vi "solenoid-sample.vi"() -> ()   [LabVIEW 2020]
uses:
  <vilib>/Rock Robotics/SystemInterfaces/DIO/FPGA_DIORelayChannel.ctl
  <vilib>/Rock Robotics/WPI/Relay/WPI_RelayDirection.ctl
  <vilib>/Rock Robotics/WPI/Relay/WPI_RelayValue.ctl
  <vilib>/Rock Robotics/WPI/Solenoid/WPI_SolenoidChannel.ctl
  <vilib>/Rock Robotics/WPI/Solenoid/WPI_SolenoidValue.ctl
  <vilib>/Rock Robotics/WPI/ThirdParty/JAS_Junk/TrajLib/Timer_New.vi
  <vilib>/Rock Robotics/WPI/Utilities/WPI_GetSetVariantRefNum.vi
  <vilib>/Rock Robotics/Network Tables/NT Write Boolean.vi
  <vilib>/Rock Robotics/Network Tables/NT Write Number.vi
  <vilib>/Rock Robotics/WPI/Solenoid/WPI_SolenoidOpenSingle.vi
  <vilib>/Rock Robotics/WPI/Solenoid/WPI_SolenoidOpenDouble.vi
  <vilib>/Rock Robotics/WPI/Solenoid/WPI_SolenoidSetEnum.vi
  <vilib>/Utility/semaphor.llb/Obtain Semaphore Reference.vi
  <vilib>/Rock Robotics/WPI/ThirdParty/JAS_Junk/TrajLib/Timer_Reset.vi
  <vilib>/Rock Robotics/WPI/ThirdParty/JAS_Junk/TrajLib/Timer_Start.vi
  <vilib>/Rock Robotics/WPI/ThirdParty/JAS_Junk/TrajLib/Timer_HasPeriodPassedOnce.vi
  <vilib>/Rock Robotics/WPI/ThirdParty/JAS_Junk/TrajLib/Timer_Stop.vi
  <vilib>/Rock Robotics/Network Tables/NT Write Integer.vi
  <vilib>/Rock Robotics/WPI/ThirdParty/JAS_Junk/TrajLib/Trajectory_Library.lvlib
panel:
  in  "ROBOT\nENABLED":bool
  in  "SOLENOID\nCONTROL":bool
  in  "SOLENOID\nCONTROL":bool
  in  "RELAY\nREVERSE":bool
  in  "RELAY\nFORWARD":bool
  in  "RELAY\nCONTROL":bool
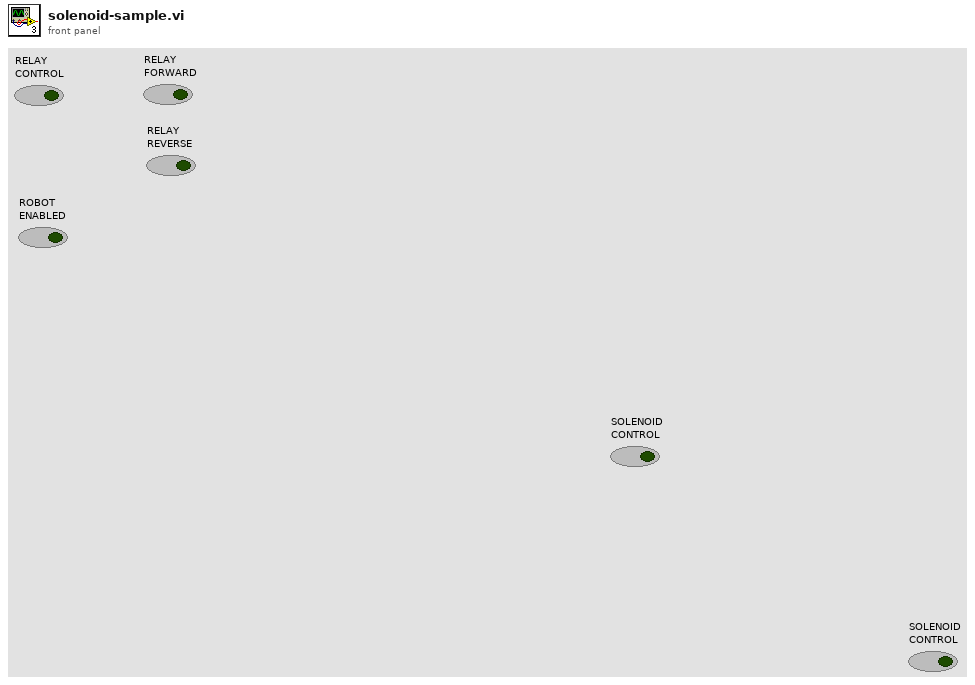
[diagram p1: front panel]
types:
  T1 = typedef "WPI_SolenoidValue.ctl" = enum16{"Off", "On", "Forward", "Reverse"}
  T2 = typedef "WPI_SolenoidChannel.ctl" = enum8{"Solenoid 0", "Solenoid 1", "Solenoid 2", "Solenoid 3", "Solenoid 4", "Solenoid 5", "Solenoid 6", "Solenoid 7", "Solenoid 8", "Solenoid 9", "Solenoid 10", "Solenoid 11", "Solenoid 12", "Solenoid 13", "Solenoid 14", "Solenoid 15", "Invalid"}
  T3 = typedef "WPI_RelayValue.ctl" = enum16{"Off", "On", "Forward", "Reverse"}
  T4 = typedef "WPI_RelayDirection.ctl" = enum16{"Both directions", "Forward only", "Reverse only"}
  T5 = typedef "FPGA_DIORelayChannel.ctl" = enum8{"Relay 0", "Relay 1", "Relay 2", "Relay 3", "Invalid"}
  T6 = typedef "WPI_CompressorDevRef.ctl" = cluster{"DevStatus":errorcluster, "Pneumatics Control Module":u8}
  T7 = typedef "WPI_RelayDevRef.ctl" = cluster{"DevStatus":errorcluster, "Relay Channel":T5, "Relay Direction":T4}
  T8 = typedef "WPI_SolenoidDevRef.ctl" = cluster{"DevStatus":errorcluster, "Pneumatics Control Module":u8, "Forward Solenoid Channel":T2, "Reverse Solenoid Channel":T2}
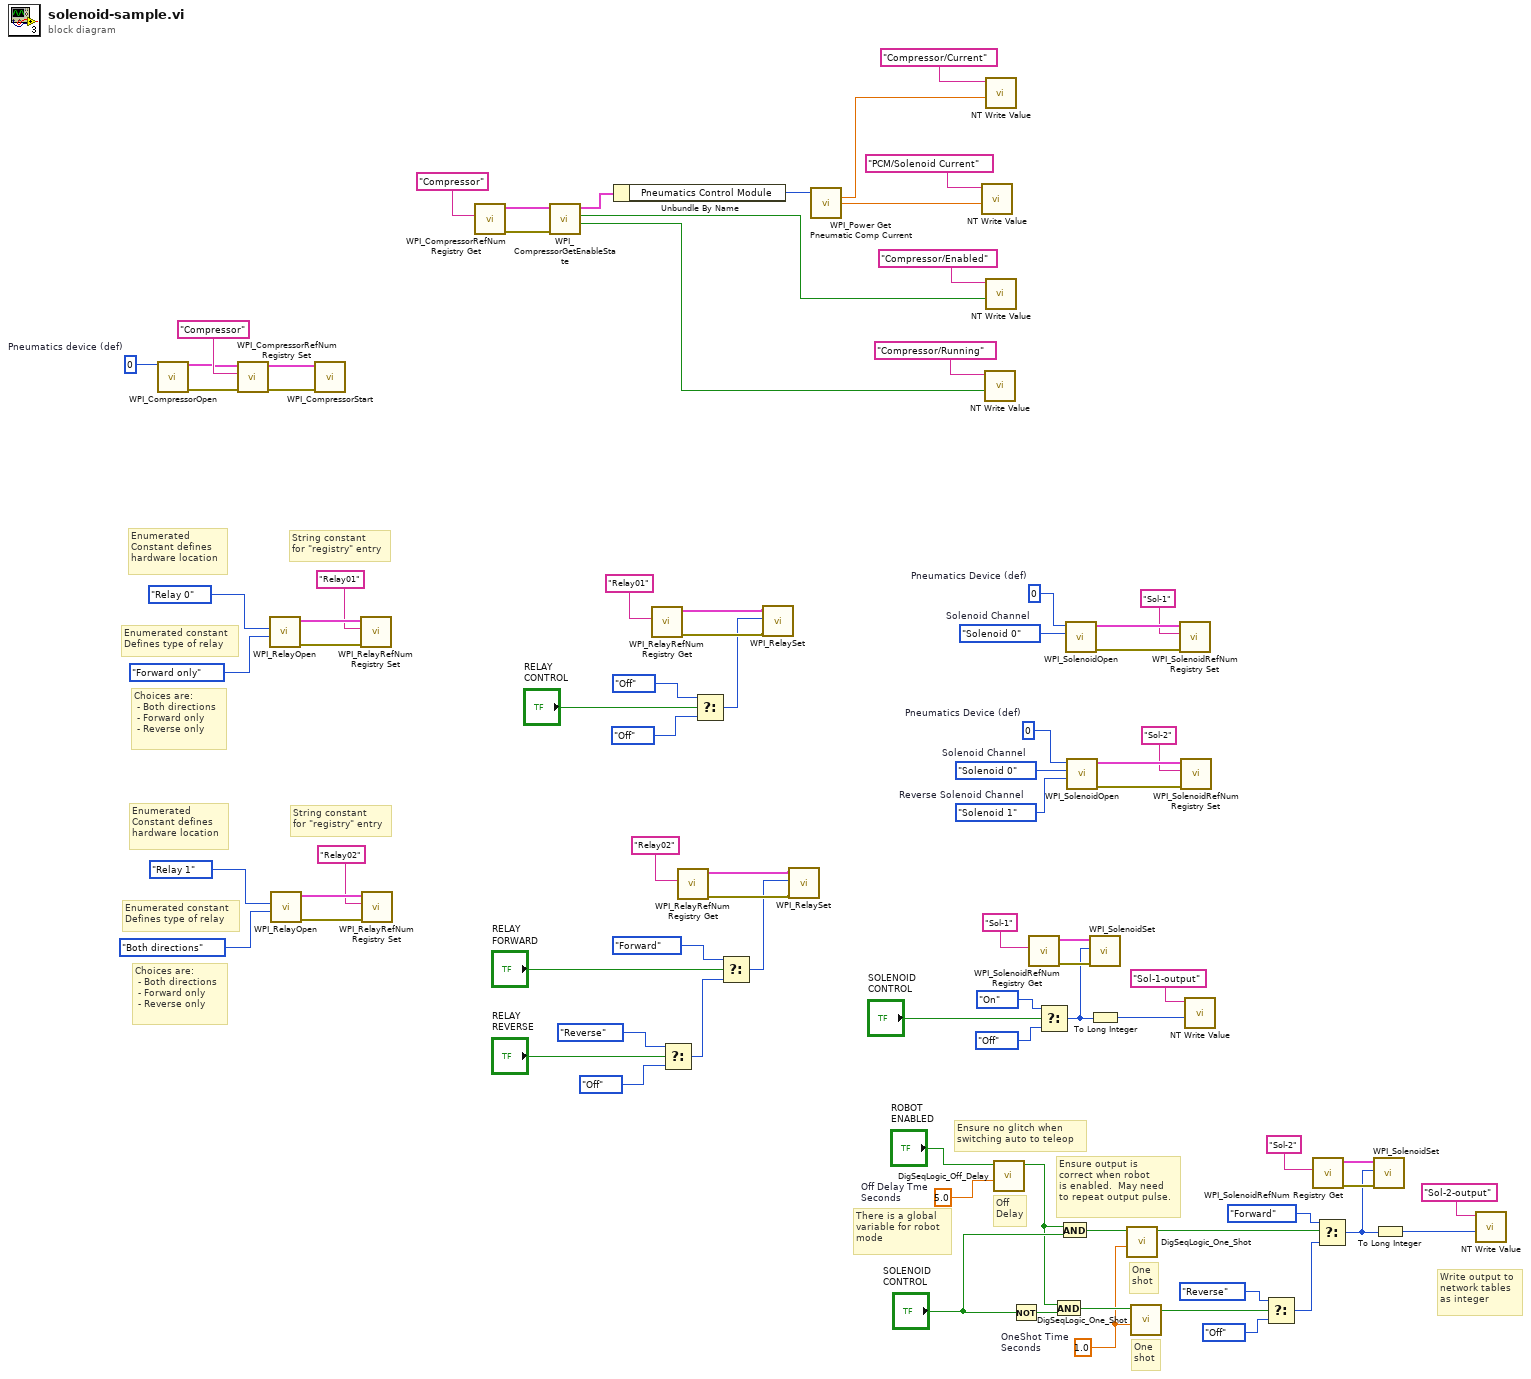
[diagram p0: block diagram]
diagram:
  w1 = 1.0  # OneShot Time Seconds
  w19 = 5.0  # Off Delay Tme Seconds
  w30 = WPI_SolenoidChannel."Solenoid 1"  # Reverse Solenoid Channel
  w31 = WPI_SolenoidChannel."Solenoid 0"  # Solenoid Channel
  w32 = u8 0  # Pneumatics Device (def)
  w36 = WPI_SolenoidChannel."Solenoid 0"  # Solenoid Channel
  w37 = u8 0  # Pneumatics Device (def)
  w59 = u8 0  # Pneumatics device (def)
  # "Ensure no glitch when\nswitching auto to teleop"
  # "There is a global \nvariable for robot \nmode"
  # "Write output to\nnetwork tables\nas integer"
  # "Ensure output is\ncorrect when robot\nis enabled.  May need\nto repeat output pulse."
  # "One \nshot"
  # "One \nshot"
  # "Off \nDelay"
  # "Choices are:\n - Both directions\n - Forward only\n - Reverse only"
  # "String constant\nfor \"registry\" entry"
  # "Enumerated constant\nDefines type of relay"
  # "Enumerated\nConstant defines\nhardware location"
  # "Choices are:\n - Both directions\n - Forward only\n - Reverse only"
  # "String constant\nfor \"registry\" entry"
  # "Enumerated constant\nDefines type of relay"
  # "Enumerated\nConstant defines\nhardware location"
  n1 = call <vilib>:"WPI_CompressorOpen.vi"("Pneumatics device (def)"=w59) -> ("CompressorDevRef"=w51:T6, "error out"=w57:errorcluster)  [unwired: 13 in]
  n2 = call <vilib>:"WPI_CompressorRefNum Registry Set.vi"("error in (no error)"=w57, "refnum name"="Compressor", "CompressorDevRef"=w51) -> ("error out"=w55:errorcluster, "CompressorDevRef"=w56:T6)  [unwired: 7 in]
  n3 = call <vilib>:"WPI_RelayOpen.vi"("Relay Direction"=WPI_RelayDirection."Forward only", "Relay Channel"=FPGA_DIORelayChannel."Relay 0") -> ("error out"=w82:errorcluster, "RelayDevRef"=w86:T7)  [unwired: 8 in]
  n4 = call <vilib>:"WPI_RelayOpen.vi"("Relay Direction"=WPI_RelayDirection."Both directions", "Relay Channel"=FPGA_DIORelayChannel."Relay 1") -> ("error out"=w77:errorcluster, "RelayDevRef"=w81:T7)  [unwired: 8 in]
  n5 = call <vilib>:"WPI_CompressorStart.vi"("error in (no error)"=w55, "CompressorDevRef"=w56) -> ()  [unwired: 8 in, 2 out]
  n6 = call <vilib>:"WPI_RelayRefNum Registry Set.vi"("error in (no error)"=w82, "refnum name"="Relay01", "RelayDevRef"=w86) -> ()  [unwired: 7 in, 2 out]
  n7 = call <vilib>:"WPI_RelayRefNum Registry Set.vi"("error in (no error)"=w77, "refnum name"="Relay02", "RelayDevRef"=w81) -> ()  [unwired: 7 in, 2 out]
  n8 = call <vilib>:"WPI_CompressorRefNum Registry Get.vi"("refnum name"="Compressor") -> ("error out"=w52:errorcluster, "CompressorDevRef"=w53:T6)  [unwired: 9 in]
  n9 = call <vilib>:"WPI_CompressorGetEnableState.vi"("error in (no error)"=w52, "CompressorDevRef"=w53) -> ("Compressor Running"=w46:bool, "Enabled"=w45:bool, "CompressorDevRef"=w50:T6)  [unwired: 3 in, 4 out]
  n10 = Unbundle By Name(w50) -> ("Pneumatics Control Module"=w49:u8)
  n11 = call <vilib>:"WPI_RelayRefNum Registry Get.vi"("refnum name"="Relay01") -> ("error out"=w75:errorcluster, "RelayDevRef"=w76:T7)  [unwired: 9 in]
  n12 = Select(t=WPI_RelayValue."Reverse" ("RelayValue"), s="RELAY\nREVERSE", f=WPI_RelayValue."Off" ("RelayValue")) -> (s? t:f=w60:T3)
  n13 = call <vilib>:"WPI_RelayRefNum Registry Get.vi"("refnum name"="Relay02") -> ("error out"=w68:errorcluster, "RelayDevRef"=w69:T7)  [unwired: 9 in]
  n14 = Select(t=WPI_RelayValue."Off" ("RelayValue"), s="RELAY\nCONTROL", f=WPI_RelayValue."Off" ("RelayValue")) -> (s? t:f=w71:T3)
  n15 = Select(t=WPI_RelayValue."Forward" ("RelayValue"), s="RELAY\nFORWARD", f=w60) -> (s? t:f=w65:T3)
  n16 = call <vilib>:"WPI_RelaySet.vi"("error in (no error)"=w75, "RelayValue"=w71, "RelayDevRef"=w76) -> ()  [unwired: 7 in, 2 out]
  n17 = call <vilib>:"WPI_RelaySet.vi"("error in (no error)"=w68, "RelayValue"=w65, "RelayDevRef"=w69) -> ()  [unwired: 7 in, 2 out]
  n18 = call <vilib>:"WPI_Power Get Pneumatic Comp Current.vi"("Pneumatics device (def)"=w49) -> ("current (A)"=w42:dbl, "Total Solenoid A"=w41:dbl)  [unwired: 12 in, 1 out]
  n19 = call-poly <vilib>:"NT Write Value.vi"("value"=w41, "name"="PCM/Solenoid Current") -> ()  [unwired: 9 in, 1 out]
  n20 = call-poly <vilib>:"NT Write Value.vi"("value"=w46, "name"="Compressor/Running") -> ()  [unwired: 9 in, 1 out]
  n21 = call-poly <vilib>:"NT Write Value.vi"("value"=w42, "name"="Compressor/Current") -> ()  [unwired: 9 in, 1 out]
  n22 = call-poly <vilib>:"NT Write Value.vi"("value"=w45, "name"="Compressor/Enabled") -> ()  [unwired: 9 in, 1 out]
  n23 = call <vilib>:"DigSeqLogic_Off_Delay.vi"("Delay"=w19, "Input"="ROBOT\nENABLED") -> ("Output"=w13:bool)  [unwired: 8 in, 1 out]
  n24 = Not(x="SOLENOID\nCONTROL") -> (.not. x?=w17:bool)
  n25 = call <vilib>:"WPI_SolenoidRefNum Registry Get.vi"("refnum name"="Sol-1") -> ("error out"=w28:errorcluster, "SolenoidDevRef"=w27:T8)  [unwired: 9 in]
  n26 = Select(t=WPI_SolenoidValue."On" ("Value"), s="SOLENOID\nCONTROL", f=WPI_SolenoidValue."Off" ("Value")) -> (s? t:f=w6:T1)
  n27 = And(x=w13, y=w17) -> (x .and. y?=w16:bool)
  n28 = And(x=w13, y="SOLENOID\nCONTROL") -> (x .and. y?=w15:bool)
  n29 = call-poly <vilib>:"WPI_SolenoidOpen.vi"("Solenoid Channel"=w36, "Pneumatics Device (def)"=w37) -> ("error out"=w39:errorcluster, "SolenoidDevRef"=w40:T8)  [unwired: 8 in]
  n30 = call-poly <vilib>:"WPI_SolenoidOpen.vi"("Reverse Solenoid Channel"=w30, "Forward Solenoid Channel"=w31, "Pneumatics Device (def)"=w32) -> ("error out"=w34:errorcluster, "SolenoidDevRef"=w35:T8)  [unwired: 7 in]
  n31 = call-poly <vilib>:"WPI_SolenoidSet.vi"("error in (no error)"=w28, "Value"=w6, "SolenoidDevRef"=w27) -> ()  [unwired: 7 in, 2 out]
  n32 = To Long Integer(number=w6) -> (32bit integer=w2:i32)
  n33 = call <vilib>:"DigSeqLogic_One_Shot.vi"("OneShot"=w1, "Input"=w15) -> ("Output"=w9:bool)  [unwired: 8 in, 1 out]
  n34 = call <vilib>:"DigSeqLogic_One_Shot.vi"("OneShot"=w1, "Input"=w16) -> ("Output"=w8:bool)  [unwired: 8 in, 1 out]
  n35 = call <vilib>:"WPI_SolenoidRefNum Registry Set.vi"("error in (no error)"=w39, "refnum name"="Sol-1", "SolenoidDevRef"=w40) -> ()  [unwired: 7 in, 2 out]
  n36 = call <vilib>:"WPI_SolenoidRefNum Registry Set.vi"("error in (no error)"=w34, "refnum name"="Sol-2", "SolenoidDevRef"=w35) -> ()  [unwired: 7 in, 2 out]
  n37 = call-poly <vilib>:"NT Write Value.vi"("value"=w2, "name"="Sol-1-output") -> ()  [unwired: 9 in, 1 out]
  n38 = Select(t=WPI_SolenoidValue."Reverse" ("Value"), s=w8, f=WPI_SolenoidValue."Off" ("Value")) -> (s? t:f=w10:T1)
  n39 = call <vilib>:"WPI_SolenoidRefNum Registry Get.vi"("refnum name"="Sol-2") -> ("error out"=w22:errorcluster, "SolenoidDevRef"=w21:T8)  [unwired: 9 in]
  n40 = Select(t=WPI_SolenoidValue."Forward" ("Value"), s=w9, f=w10) -> (s? t:f=w7:T1)
  n41 = call-poly <vilib>:"WPI_SolenoidSet.vi"("error in (no error)"=w22, "Value"=w7, "SolenoidDevRef"=w21) -> ()  [unwired: 7 in, 2 out]
  n42 = To Long Integer(number=w7) -> (32bit integer=w4:i32)
  n43 = call-poly <vilib>:"NT Write Value.vi"("value"=w4, "name"="Sol-2-output") -> ()  [unwired: 9 in, 1 out]
